vi "FILE_DIALOG 2016.vi"(0 "flow_slope_IN":dbl=51.35 format="%.2f", 1 "pressure_slope_IN":dbl=23.33 format="%.2f", 3 "string_pot_slope_IN":dbl=1.5 format="%.2f", 4 "Descriptions":string[](array[string]), 5 "error in (no error)":errorcluster, 6 "start path":path=path "D:/Cascade/Data/Output Files", 7 "Sensor Cluster":T1, 10 "Array in":refnum<k24>[](array[refnum])) -> (8 "path":path, 9 "Sensor Cluster 2":T1, 11 "exists":bool, 12 "Array out":refnum<k24>[](array[refnum]), 14 "flow_slope_OUT":dbl=51.35 format="%.2f", 15 "pressure_slope_OUT":dbl=732.5347533511234 format="%.2f", 17 "string_pot_slope_OUT":dbl=1.5 format="%.2f", 19 "error out":errorcluster)   [LabVIEW 2016]
uses:
  C:/Program Files (x86)/National Instruments/LabVIEW 2016/vi.lib/ULx/ULx_LV.dll
  Waterloo DAQ/controls/MCC DAQ Readings.ctl
panel:
  out "cal_completed":bool
  out "new_or _prev_file_selected":bool
  in  "calibrate_KPRO":bool
  in  "previous_file":bool
  in  "new_file":bool
  in  "OK Button":bool
  # "Select root file\nsuch as test.csv"
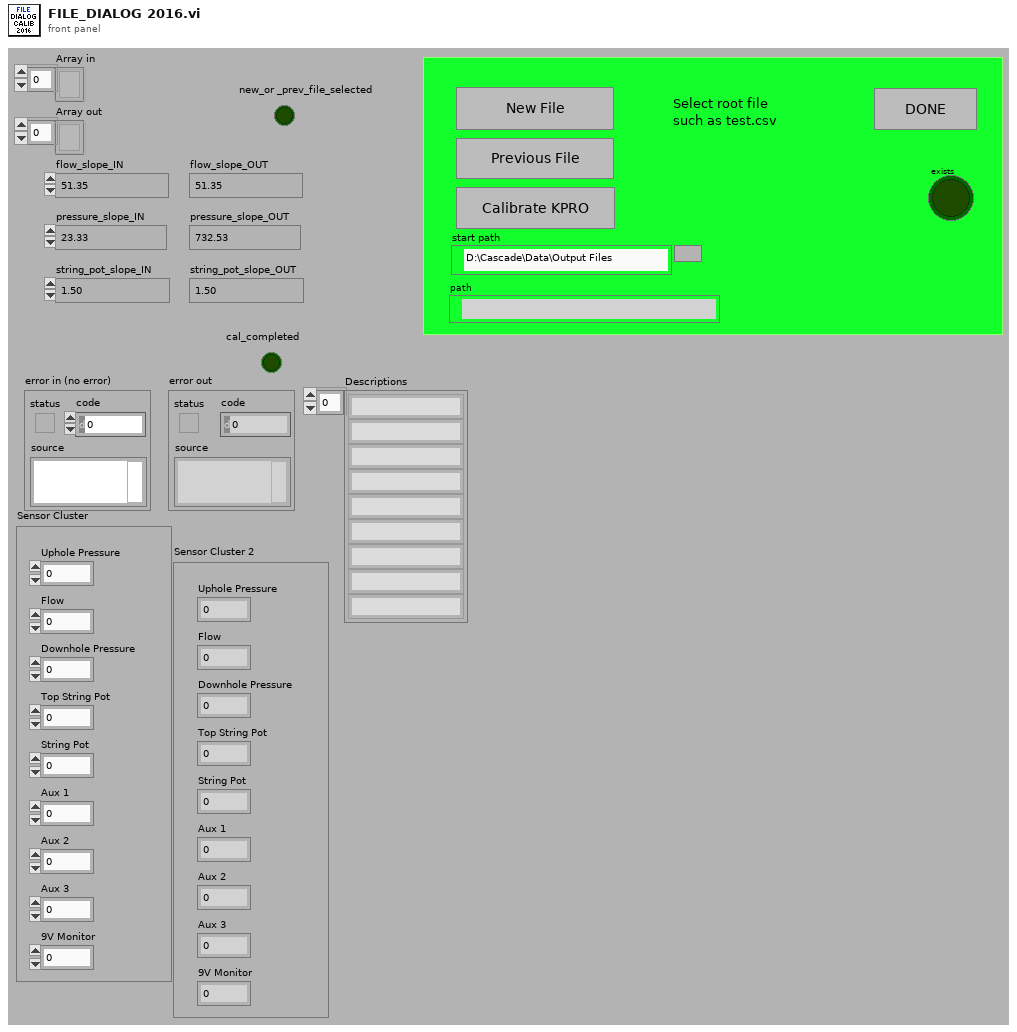
[diagram p1: front panel]
types:
  T1 = typedef "MCC DAQ Readings.ctl" = cluster{"Uphole Pressure":dbl, "Flow":dbl, "Downhole Pressure":dbl, "Top String Pot":dbl, "String Pot":dbl, "Aux 1":dbl, "Aux 2":dbl, "Aux 3":dbl, "9V Monitor":dbl}
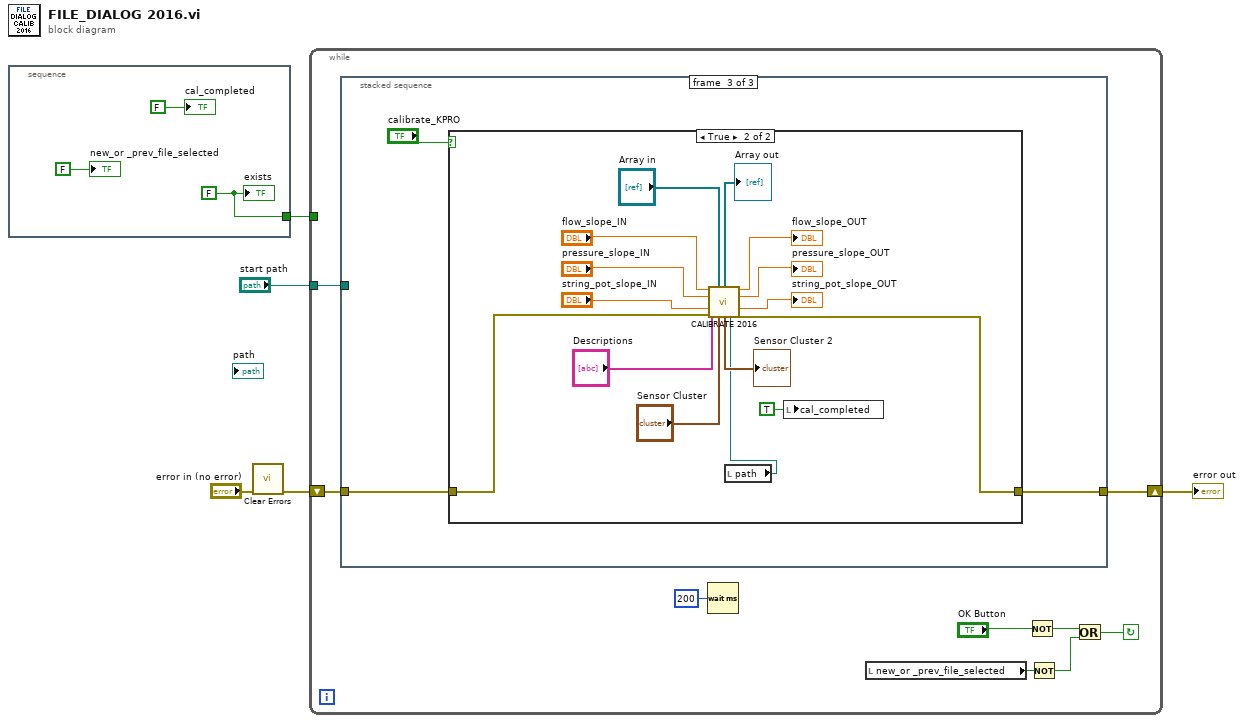
[diagram p0: block diagram]
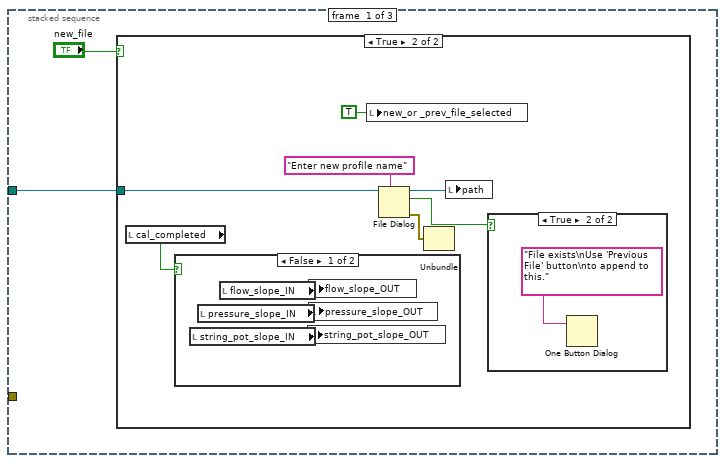
[diagram p2: hidden frame]
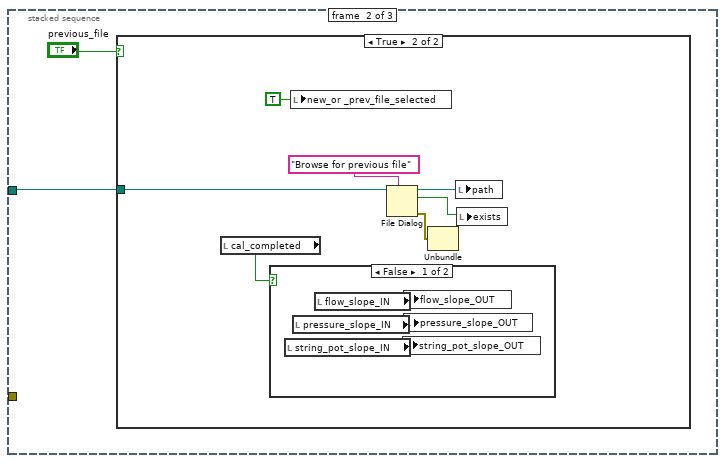
[diagram p6: hidden frame]
diagram:
  n1 = stacked-sequence {
    tunnel: [w8] -> w5
    frame #0 {
      w8 = FALSE ("exists")
      "exists" <- w8
      "new_or _prev_file_selected" <- FALSE ("new_or _prev_file_selected")
      "cal_completed" <- FALSE ("cal_completed")
    }
  }
  n2 = call <vilib>:"Clear Errors.vi"("error in (no error)"="error in (no error)") -> ("error out"=w1:errorcluster)  [unwired: 5 in, 1 out]
  n3 = while {
    shift-left: w1 -> [w14]
    shift-right: [w13] -> w2
    tunnel: "start path" -> [w15]
    tunnel: w5 -> [_]
    stop <- w12 continue-if-true
    n4 = stacked-sequence {
      tunnel: w15 -> [w18 w31 _]
      tunnel: w14 -> [_ _ w44]
      tunnel: [_ _ w43] -> w13
      frame #0 {
        n5 = case shown="True" "new_file" {
          tunnel: w18 -> [_ w23]
          frame False {
          }
          frame True {
            n6 = local read "cal_completed"() -> (w21:bool)
            n7 = case shown="False" w21 {
              frame False {
                n8 = local read "string_pot_slope_IN"() -> (w27:dbl)
                n9 = local read "pressure_slope_IN"() -> (w28:dbl)
                n10 = local read "flow_slope_IN"() -> (w29:dbl)
                n11 = local write "string_pot_slope_OUT"(w27) -> ()
                n12 = local write "flow_slope_OUT"(w29) -> ()
                n13 = local write "pressure_slope_OUT"(w28) -> ()
              }
              frame True {
              }
            }
            n14 = local write "new_or _prev_file_selected"(TRUE ("new_or _prev_file_selected")) -> ()
            n15 = File Dialog(7:"Enter new profile name" ("prompt"), 11:w23) -> (0:w20:errorcluster, 2:w24:bool, 3:w25:path)  [unwired: 5 in, 1 out]
            n16 = Unbundle(w20) -> ()  [unwired: 3 out]
            n17 = local write "path"(w25) -> ()
            n18 = case shown="True" w24 {
              frame False {
              }
              frame True {
                n19 = One Button Dialog(message="File exists\nUse 'Previous File' button\nto append to this.") -> ()  [unwired: 1 in, 1 out]
              }
            }
          }
        }
      }
      frame #1 {
        n20 = case shown="True" "previous_file" {
          tunnel: w31 -> [_ w36]
          frame False {
          }
          frame True {
            n21 = local read "cal_completed"() -> (w34:bool)
            n22 = case shown="False" w34 {
              frame False {
                n23 = local read "string_pot_slope_IN"() -> (w40:dbl)
                n24 = local read "pressure_slope_IN"() -> (w41:dbl)
                n25 = local read "flow_slope_IN"() -> (w42:dbl)
                n26 = local write "string_pot_slope_OUT"(w40) -> ()
                n27 = local write "flow_slope_OUT"(w42) -> ()
                n28 = local write "pressure_slope_OUT"(w41) -> ()
              }
              frame True {
              }
            }
            n29 = local write "new_or _prev_file_selected"(TRUE ("new_or _prev_file_selected")) -> ()
            n30 = File Dialog(7:"Browse for previous file" ("prompt"), 11:w36) -> (0:w33:errorcluster, 2:w37:bool, 3:w38:path)  [unwired: 5 in, 1 out]
            n31 = Unbundle(w33) -> ()  [unwired: 3 out]
            n32 = local write "path"(w38) -> ()
            n33 = local write "exists"(w37) -> ()
          }
        }
      }
      frame #2 {
        n34 = case shown="True" "calibrate_KPRO" {
          tunnel: w44 -> [w46 w58]
          tunnel: [w46 w57] -> w43
          frame False {
          }
          frame True {
            n35 = local read "path"() -> (w47:path)
            n36 = call "CALIBRATE 2016.vi"("flow_slope_IN"="flow_slope_IN", "Array in"="Array in", "pressure_slope_IN"="pressure_slope_IN", "Descriptions"="Descriptions", "string_pot_slope_IN"="string_pot_slope_IN", "error in (no error)"=w58, "Sensor Cluster"="Sensor Cluster", "Path"=w47) -> ("Array out"=→"Array out":refnum<k24>[], "flow_slope_OUT"=→"flow_slope_OUT":dbl, "pressure_slope_OUT"=→"pressure_slope_OUT":dbl, "string_pot_slope_OUT"=→"string_pot_slope_OUT":dbl, "Sensor Cluster 2"=→"Sensor Cluster 2":T1, "error out"=w57:errorcluster)  [unwired: 2 in]
            n37 = local write "cal_completed"(TRUE ("cal_completed")) -> ()
          }
        }
      }
    }
    n38 = Wait (ms)(milliseconds to wait=u32 200) -> ()  [unwired: 1 out]
    n39 = local read "new_or _prev_file_selected"() -> (w10:bool)
    n40 = Not(x="OK Button") -> (.not. x?=w11:bool)
    n41 = Not(x=w10) -> (.not. x?=w9:bool)
    n42 = Or(x=w11, y=w9) -> (x .or. y?=w12:bool)
  }
  "error out" <- w2
